vi "Main_05a.vi"() -> ()   [LabVIEW 2023]
uses:
  ENUM_Ranges.ctl
  MAP_Connections.ctl
  ENUM_map names.ctl
  Cluster_Sorce Destination Connection.ctl
  <vilib>/Utility/miscctls.llb/LVMapReplaceAction.ctl
  d4d7e510-1f78-48c4-9a23-25f0a9fbcbc6.vi
panel:
  out "answer":i64
  out "Connections":T1
  out "Seed array":i64[](array[numeric])
  out "array w/ subset deleted":string[](array[string])
  in  "Ranges":T4
  out "Answer":u32
  in  "Puzzle":string="seeds: 3416930225 56865175 4245248379 7142355 1808166864 294882110 863761171 233338109 4114335326 67911591 1198254212 504239157 3491380151 178996923 3965970270 15230597 2461206486 133606394 2313929258 84595688\n\nseed-to-soil map:\n3534435790 4123267198 50004089\n3584439879 3602712894 238659237\n2263758314 0 160870825\n2971481857 2850687195 31776688\n4173604159 3353763588 121363137\n3823099116 3003258545 350505043\n2850687195 2882463883 120794662\n1503174517 2076905328 347723811\n1850898328 195477286 412859986\n1265521310 1606247567 17062682\n3285153612 4173271287 121696009\n488201540 828927797 777319770\n453595079 160870825 34606461\n3406849621 3475126725 127586169\n1282583992 608337272 220590525\n3003258545 3841372131 281895067\n0 1623310249 453595079\n\nsoil-to-fertilizer map:\n131427930 1185330183 180485664\n748806267 2475960003 160820884\n311913594 3858074623 436892673\n3738185633 2255483282 220476721\n909627151 2636780887 1221293736\n2848518198 1365815847 889667435\n2130920887 131427930 666553095\n2797473982 1134285967 51044216\n3958662354 797981025 336304942\n\nfertilizer-to-water map:\n318410581 1095359367 168721315\n1850530626 4267113166 11515024\n1868157768 2129267011 114327162\n3662276437 4191001581 22313216\n2980811924 3765310336 180818294\n3971289879 3991326516 15449292\n4217905563 2279561459 35118050\n2287003279 4213314797 47187938\n1837473204 2314679509 13057422\n1998824036 3946128630 45197886\n222462505 1264080682 95948076\n487131896 791770420 303588947\n4253023613 4068573955 41943683\n2334191217 3252696905 278223677\n3986739171 2786104784 83568826\n3495640623 3600917310 61383314\n3557023937 3662300624 15042395\n2222048360 3535962391 64954919\n2919013777 4006775808 61798147\n3660033649 4182646675 2242788\n3266573705 2327736931 229066918\n3684589653 2869673610 235425729\n3261531896 3530920582 5041809\n790720843 417781090 105163807\n895884650 0 159434487\n2044021922 2608078346 178026438\n1862045650 4184889463 6112118\n3572066332 3677343019 87967317\n1830862773 4260502735 6610431\n1338009275 159434487 258346603\n3233759255 1830862773 27772641\n1055319137 1360028758 282690138\n1982484930 4278628190 16339106\n2883046491 2243594173 35967286\n2612414894 1858635414 270631597\n4070307997 3105099339 147597566\n3161630218 4110517638 72129037\n1596355878 522944897 46363018\n0 569307915 222462505\n3920015382 2556803849 51274497\n\nwater-to-light map:\n3185219492 1324735395 185266775\n3146586681 1249776213 38632811\n28244350 428471809 312696716\n340941066 3650819202 117391304\n458332370 963661621 286114592\n2785969088 3483794777 117695215\n1279106820 1583617352 194624401\n1473731221 3601489992 49329210\n0 2796264154 28244350\n744446962 3356330358 127464419\n2562107674 223281414 205190395\n3544929092 0 223281414\n2767298069 944990602 18671019\n2903664303 775683406 169307196\n3072971499 1510002170 73615182\n1140236238 741168525 34514881\n1242780449 1288409024 36326371\n1523060431 1778241753 949993071\n871911381 3088005501 268324857\n3370486267 2913562676 174442825\n4096117687 4180659844 114307452\n1174751119 2728234824 68029330\n4210425139 4096117687 84542157\n2473053502 2824508504 89054172\n\nlight-to-temperature map:\n57304962 1726059676 351776583\n1567802332 965133212 510033927\n3296678005 3095070487 435408435\n2476702913 3609026358 293401880\n1363411758 0 204390574\n1017340727 204390574 346071031\n2770104793 2148583721 409359530\n994650876 1475167139 22689851\n0 550461605 20445762\n20445762 1692752937 33306739\n2144982382 2092188566 56395155\n799754929 1497856990 194895947\n53752501 961580751 3552461\n409081545 570907367 390673384\n2201377537 3902428238 275325376\n3988154754 2557943251 306812542\n3179464323 4177753614 117213682\n3732086440 3530478922 78547436\n3810633876 2864755793 177520878\n2092188566 3042276671 52793816\n\ntemperature-to-humidity map:\n18928354 3414191527 36074961\n3774151818 3588716061 144651966\n2046448856 1384376044 7569690\n2737178317 903028814 27883660\n2981004508 930912474 349046239\n1609626976 3084565214 120015958\n2765061977 2248931514 215942531\n157942811 3887783726 359543023\n3330050747 2195105292 25002873\n2041971091 78356652 4477765\n1938796124 861459710 41569104\n1608860129 2474627144 766847\n1812604664 3795542966 74143188\n4196563819 3386335999 27024746\n1980365228 3204581172 61605863\n1136292153 82834417 94266783\n4015908448 1279958713 104417331\n2701246339 2062523244 35931978\n4223588565 3286123619 23738184\n91521115 3309861803 56668597\n1886747852 2552562071 52048272\n1729642934 0 61644451\n1791287385 1504576228 21317279\n517485834 1726582276 261020280\n2192468119 2604610343 479954871\n1413642666 1391945734 112630494\n71715516 3366530400 19805599\n3918803784 2475393991 77168080\n1546685190 3733368027 62174939\n2672422990 2220108165 28823349\n148189712 2464874045 9753099\n18097572 3413360745 830782\n0 3869686154 18097572\n3995971864 3266187035 19936584\n853426802 432206724 27759827\n2054018546 3450266488 138449573\n881186629 177101200 255105524\n778506114 1987602556 74920688\n1526273160 2098455222 20412030\n55003315 61644451 16712201\n3355053620 459966551 401493159\n4120325779 2118867252 76238040\n1230558936 1525893507 183083730\n3756546779 1708977237 17605039\n\nhumidity-to-location map:\n166973311 827072705 21017988\n2420657564 1797988486 98294592\n3711057743 1724407580 50543704\n151140540 331672683 15832771\n2611368935 1098267426 35837870\n329110209 0 39413233\n848395356 3293184115 2008343\n850403699 1508109908 216297672\n3203490893 3278069000 15115115\n1322210923 4179894531 115072765\n3761601447 848395356 249872070\n230668724 39413233 27530262\n1437283688 2240143464 113813014\n1551096702 2957294790 77256502\n716039283 695021295 132051410\n258198986 109620920 70911223\n1314022212 2357817442 8188711\n2793895840 2474472017 281155944\n385486933 347505454 330552350\n3218606008 3561131747 206517169\n1066701371 3354107909 156810008\n4011473517 1134105296 283493779\n0 180532143 151140540\n368523442 678057804 16963491\n1223511379 1417599075 90510833\n3183517648 1988699857 19973245\n2270463718 4038012896 141881635\n1817187310 1774951284 23037202\n1963899457 2755627961 201666829\n2412345353 3295192458 8312211\n1840224512 3767648916 123674945\n187991299 66943495 42677425\n2518952156 1896283078 92416779\n1628353204 3034551292 138620276\n3075051784 2366006153 108465864\n3660454503 3303504669 50603240\n3425123177 2008673102 231470362\n3656593539 2353956478 3860964\n1766973480 3510917917 50213830\n2647206805 3891323861 146689035\n2165566286 3173171568 104897432"
  in  "Example":string="seeds: 79 14 55 13\n\nseed-to-soil map:\n50 98 2\n52 50 48\n\nsoil-to-fertilizer map:\n0 15 37\n37 52 2\n39 0 15\n\nfertilizer-to-water map:\n49 53 8\n0 11 42\n42 0 7\n57 7 4\n\nwater-to-light map:\n88 18 7\n18 25 70\n\nlight-to-temperature map:\n45 77 23\n81 45 19\n68 64 13\n\ntemperature-to-humidity map:\n0 69 1\n1 0 69\n\nhumidity-to-location map:\n60 56 37\n56 93 4"
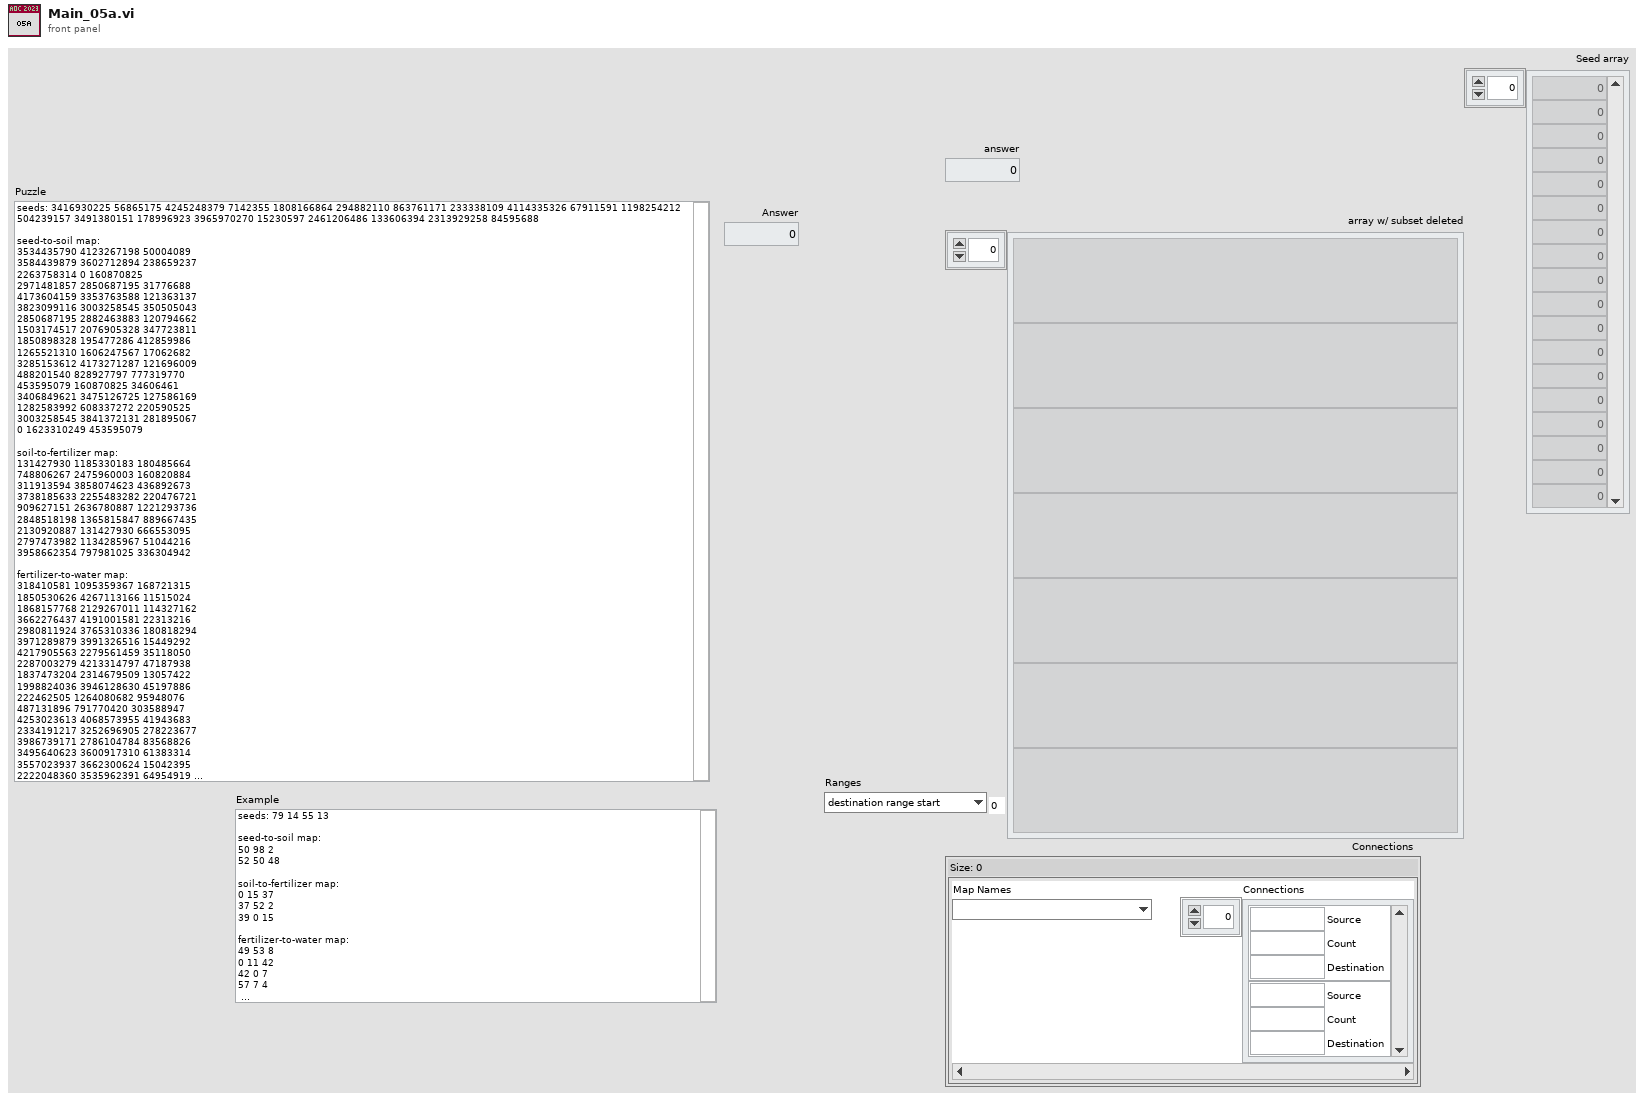
[diagram p1: front panel]
types:
  T1 = typedef "MAP_Connections.ctl" = map{T2, T3[]}
  T2 = typedef "ENUM_map names.ctl" = enum16{"seed-to-soil map:", "soil-to-fertilizer map:", "fertilizer-to-water map:", "water-to-light map:", "light-to-temperature map:", "temperature-to-humidity map:", "humidity-to-location map:"}
  T3 = typedef "Cluster_Sorce Destination Connection.ctl" = cluster{"Source":i64, "Count":i64, "Destination":i64}
  T4 = typedef "ENUM_Ranges.ctl" = enum16{"destination range start", "source range start", "range legnth"}
  T5 = typedef "LVMapReplaceAction.ctl" = enum32{"Modify Entry only if found", "Add or Modify Entry", "Delete Entry"}
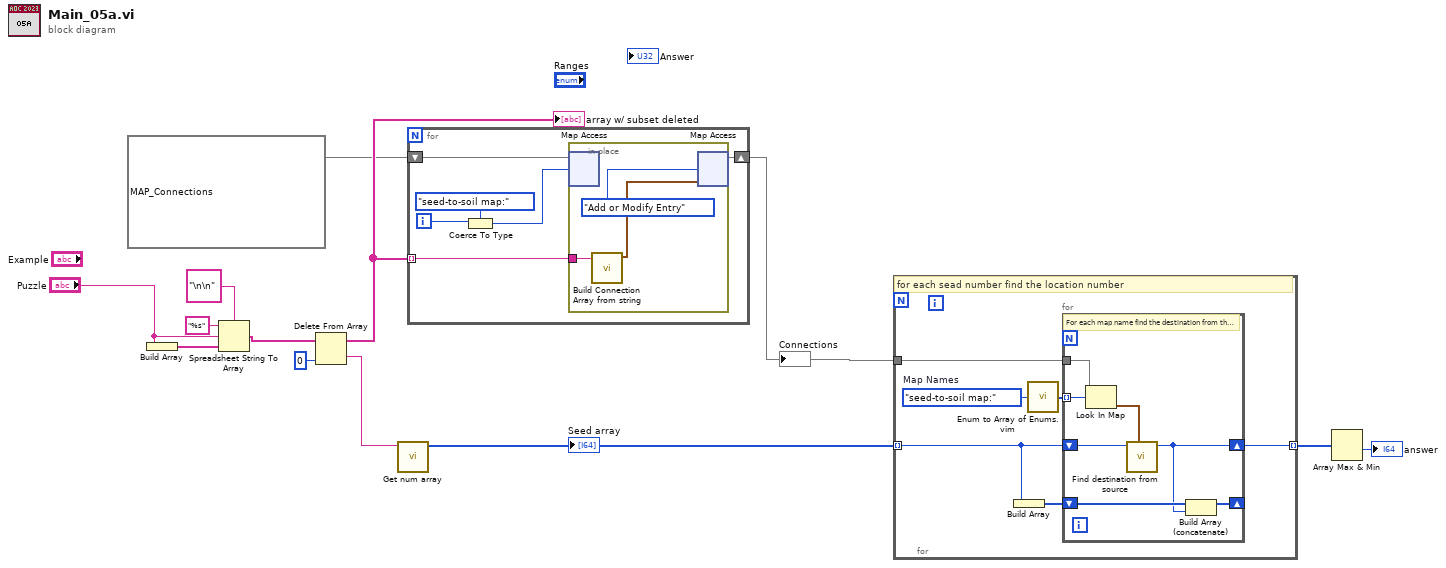
[diagram p0: block diagram]
diagram:
  n1 = Build Array("Puzzle") -> (w13:string[])
  n2 = Spreadsheet String To Array(delimiter (Tab)="\n\n", format string="%s", spreadsheet string="Puzzle", array type (2D Dbl)=w13) -> (array=w10:string[])
  n3 = Delete From Array(array=w10, index=0) -> (deleted portion=w8:string, array with subset deleted=w7:string[])  [unwired: 1 in]
  "array w/ subset deleted" <- w7
  n4 = call "Get num array.vi"("number String"=w8) -> ("number Array"=w5:i64[])  [unwired: 10 in]
  "Seed array" <- w5
  n5 = for {
    tunnel: w7 -> [w19] mode=indexing
    shift-right: [w14] -> w4
    shift-left: T1 {} ("Connections") -> [w18]
    i -> [w17]
    n6 = Coerce To Type(0:w17, 1:ENUM_map_names."seed-to-soil map:" ("Map Names")) -> (2:w15:T2)
    n7 = in-place {
      in-place-border: w19 -> [w22]
      n8 = in-place-map #1(w18, w15) -> ()  [unwired: 1 in, 2 out]
      n9 = call "Build Connection Array from string.vi"("Connection String"=w22) -> ("Range Cluster"=w21:T3[])  [unwired: 10 in]
      n10 = in-place-map #1(w21, LVMapReplaceAction."Add or Modify Entry" ("action")) -> (w14:T1)  [unwired: 2 out]
    }
  }
  "Connections" <- w4
  n11 = for {
    tunnel: w5 -> [w25] mode=indexing
    tunnel: w4 -> [w26]
    tunnel: [w23] -> w3 mode=indexing
    w28 = ENUM_map_names."seed-to-soil map:"  # Map Names
    # "for each sead number find the location number"
    n12 = Build Array(w25) -> (w24:i64[])
    n13 = call "Enum to Array of Enums.vim"("enum"=w28) -> ("array of enums"=w27:T2[])
    n14 = for {
      shift-right: [w29] -> w23
      shift-left: w25 -> [w32]
      tunnel: w27 -> [w35] mode=indexing
      tunnel: w26 -> [w34]
      shift-right: [w30] -> _
      shift-left: w24 -> [w31]
      # "For each map name find the destination from the source number"
      n15 = Look In Map(map=w34, key=w35) -> (value=w33:T3[])  [unwired: 1 in, 1 out]
      n16 = call "Find destination from source.vi"("Connections"=w33, "Source"=w32) -> ("Destination"=w29:i64)  [unwired: 8 in, 1 out]
      n17 = Build Array (concatenate)(w31, w29) -> (w30:i64[])
    }
  }
  n18 = Array Max & Min(array=w3) -> (min value=→"answer":i64)  [unwired: 3 out]
